vi "Main.vi"() -> ()   [LabVIEW 2020]
uses:
  _controls/_VIWiresData.ctl
  _queue/QueueData.ctl
  _queue/State.ctl
panel:
  in  "Info2 2":string="Step 3: Enjoy!\nLength in cm is calculated assuming 1cm = 16 pixels."
  out "Total wires length (m)":dbl format="%.2f"
  out "Total wires length (pix)":dbl
  in  "Info2":string="Step 2: Calculate wires length!\nNote: For a large number of VIs calculations might take a while!"
  in  "Info1":string="Step 1: Load VIs from folder or project"
  in  "CalculateLength":bool
  out "Number of VIs":i32
  out "VIsData":T1[](array[typedef])
  in  "Stop":bool
  in  "SelectProject":bool
  in  "SelectFolder":bool
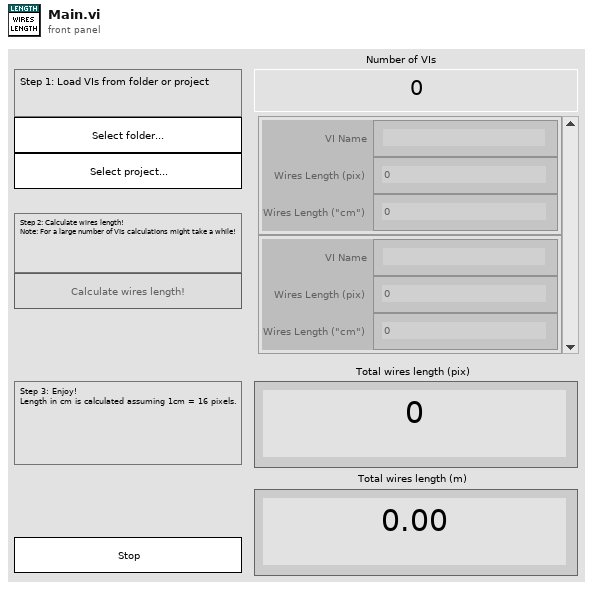
[diagram p1: front panel]
types:
  T1 = typedef "_VIWiresData.ctl" = cluster{"VI Name":string, "Wires Length (pix)":dbl, "Wires Length (\"cm\")":dbl}
  T2 = typedef "QueueData.ctl" = cluster{"State":T3, "Data":variant}
  T3 = typedef "State.ctl" = enum16{"Stop", "LoadFromFolder", "LoadFromProject", "ProcessVIsNames", "AnalyzeVIs"}
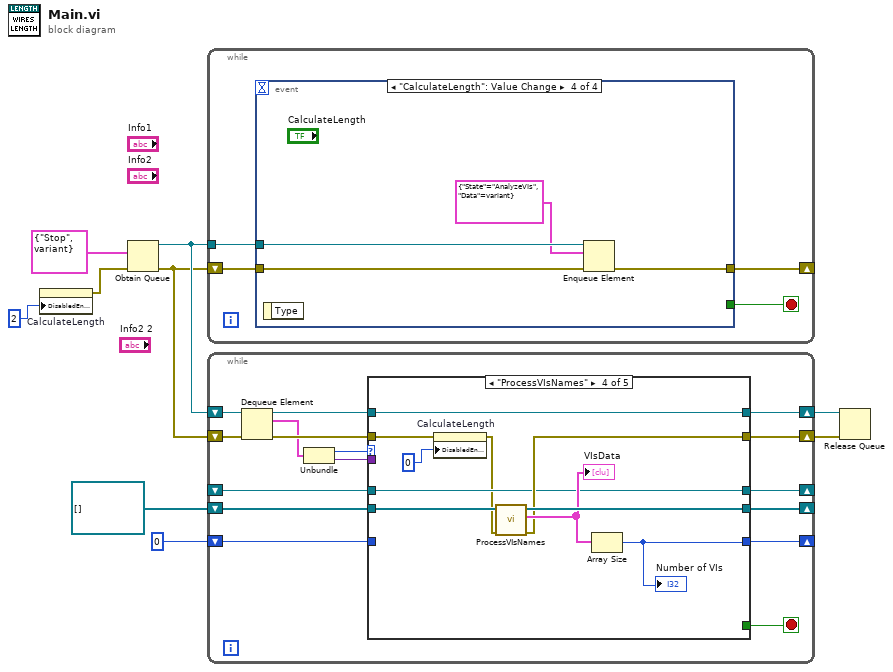
[diagram p0: block diagram]
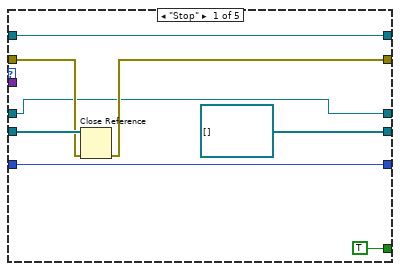
[diagram p2: hidden frame]
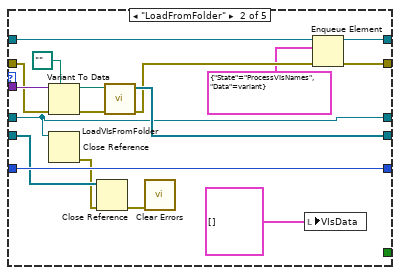
[diagram p3: hidden frame]
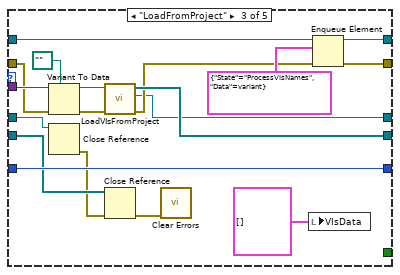
[diagram p4: hidden frame]
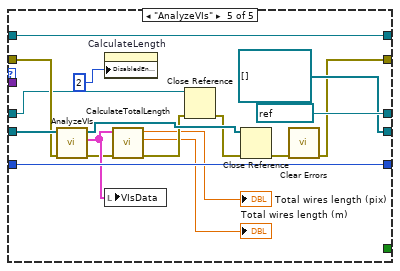
[diagram p5: hidden frame]
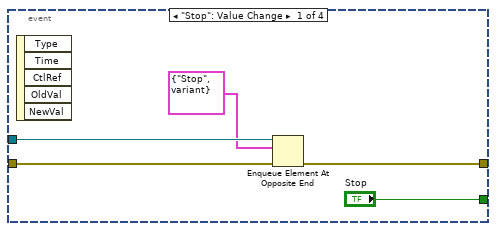
[diagram p6: hidden frame]
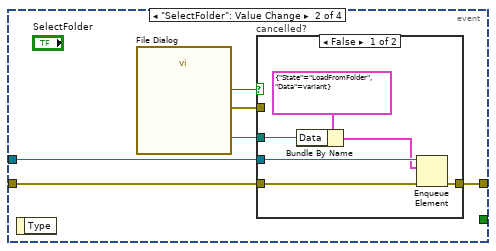
[diagram p7: hidden frame]
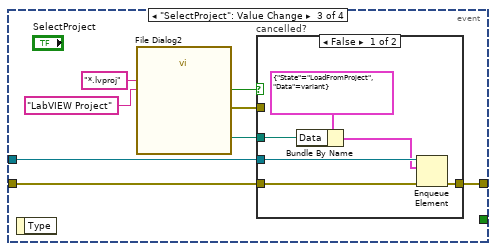
[diagram p9: hidden frame]
diagram:
  n1 = property on="CalculateLength" class="Bool"("DisabledEnum"=2) -> (error out=w1:errorcluster)  [unwired: 2 in, 1 out]
  n2 = Obtain Queue(element data type=T2 {"State"=enum."Stop", "Data"=variant} ("QueueData"), error in (no error)=w1) -> (queue out=w8:refnum<queue>, error out=w7:errorcluster)  [unwired: 3 in, 1 out]
  n3 = while {
    tunnel: w8 -> [w12]
    shift-right: [w10] -> _
    shift-left: w7 -> [w11]
    stop <- w13 stop-if-true
    n4 = event shown="[3] \"CalculateLength\": Value Change" {
      selector: _ -> [_ _ _ _]
      dyn-events: _ -> [_ _ _ _]
      timeout: _ -> [_ _ _ _]
      tunnel: ["Stop" _ _ _] -> w13
      tunnel: w12 -> [w15 w22 w37 w48]
      tunnel: w11 -> [w17 w24 w39 w50]
      tunnel: [w16 w23 w38 w49] -> w10
      event "Stop": Value Change {
        n5 = event-data() -> ()  [unwired: 1 in, 5 out]
        n6 = Enqueue Element At Opposite End(queue=w15, element=T2 {"State"=enum."Stop", "Data"=variant}, error in (no error)=w17) -> (error out=w16:errorcluster)  [unwired: 1 in, 2 out]
      }
      event "SelectFolder": Value Change {
        n7 = event-data() -> ()  [unwired: 1 in, 1 out]
        n8 = call "File Dialog"() -> ("selected path"=w21:path, "cancelled"=w20:bool, "error out"=w19:errorcluster)  [unwired: 12 in, 1 out]
        n9 = case "cancelled?" shown="False" w20 {
          tunnel: w24 -> [w30 w31]
          tunnel: [w29 w31] -> w23
          tunnel: w22 -> [w28 _]
          tunnel: w21 -> [w26 _]
          tunnel: w19 -> [_ _]
          frame False {
            n10 = Bundle By Name(cluster=T2 {"State"=enum."LoadFromFolder", "Data"=variant} ("element"), "Data"=w26) -> (w25:T2)
            n11 = Enqueue Element(queue=w28, element=w25, error in (no error)=w30) -> (error out=w29:errorcluster)  [unwired: 1 in, 2 out]
          }
          frame True {
          }
        }
      }
      event "SelectProject": Value Change {
        n12 = event-data() -> ()  [unwired: 1 in, 1 out]
        n13 = call "File Dialog2"("pattern (all files)"="*.lvproj", "pattern label"="LabVIEW Project") -> ("selected path"=w36:path, "cancelled"=w35:bool, "error out"=w33:errorcluster)  [unwired: 10 in, 1 out]
        n14 = case "cancelled?" shown="False" w35 {
          tunnel: w39 -> [w45 w46]
          tunnel: [w44 w46] -> w38
          tunnel: w37 -> [w43 _]
          tunnel: w36 -> [w41 _]
          tunnel: w33 -> [_ _]
          frame False {
            n15 = Bundle By Name(cluster=T2 {"State"=enum."LoadFromProject", "Data"=variant} ("element"), "Data"=w41) -> (w40:T2)
            n16 = Enqueue Element(queue=w43, element=w40, error in (no error)=w45) -> (error out=w44:errorcluster)  [unwired: 1 in, 2 out]
          }
          frame True {
          }
        }
      }
      event "CalculateLength": Value Change {
        n17 = event-data() -> ()  [unwired: 1 in, 1 out]
        n18 = Enqueue Element(queue=w48, element=T2 {"State"=enum."AnalyzeVIs", "Data"=variant}, error in (no error)=w50) -> (error out=w49:errorcluster)  [unwired: 1 in, 2 out]
      }
    }
  }
  n19 = while {
    shift-right: [w59] -> w6
    shift-left: w7 -> [w65]
    shift-right: [w57] -> w5
    shift-left: w8 -> [w66]
    shift-right: [w56] -> _
    shift-left: refnum<vi>[] [] ("VIs out") -> [w55]
    shift-right: [w54] -> _
    shift-left: 0 -> [w53]
    shift-right: [w52] -> _
    shift-left: _ -> [w51]
    stop <- w58 stop-if-true
    n20 = Dequeue Element(queue=w66, error in (no error)=w65) -> (queue out=w64:refnum<queue>, element=w62:T2, error out=w63:errorcluster)  [unwired: 1 in, 1 out]
    n21 = Unbundle(w62) -> ("State"=w61:T3, "Data"=w60:variant)
    n22 = case shown="\"ProcessVIsNames\"" w61 {
      tunnel: w64 -> [w73 w85 w102 w115 w136]
      tunnel: w63 -> [w71 w90 w108 w112 w133]
      tunnel: w60 -> [_ w91 w109 _ _]
      tunnel: [w70 w83 w99 w116 w120] -> w59
      tunnel: [TRUE _ _ _ _] -> w58
      tunnel: [w73 w82 w101 w115 w136] -> w57
      tunnel: [refnum<vi>[] [] ("VIs") w86 w104 w118 refnum<vi>[] [] ("VIs out")] -> w56
      tunnel: w55 -> [w72 w77 w94 w119 w134]
      tunnel: [w68 w80 w98 w114 w135] -> w54
      tunnel: w53 -> [w68 w80 w98 _ w135]
      tunnel: [w67 w78 w96 w113 refnum<vi> refnum ("Project")] -> w52
      tunnel: w51 -> [w67 w78 w95 w113 w131]
      frame "Stop" {
        n23 = Close Reference(reference=w72, error in (no error)=w71) -> (error out=w70:errorcluster)
      }
      frame "LoadFromFolder" {
        n24 = Variant To Data(error in=w90, type=path "", Variant=w91) -> (data=w88:path, error out=w87:errorcluster)
        n25 = Close Reference(reference=w78) -> (error out=w76:errorcluster)  [unwired: 1 in]
        n26 = Close Reference(reference=w77, error in (no error)=w76) -> (error out=w75:errorcluster)
        n27 = call "LoadVIsFromFolder.vi"("error in (no error)"=w87, "FolderPath"=w88) -> ("error out"=w84:errorcluster, "VIs"=w86:refnum<vi>[])  [unwired: 8 in]
        n28 = call <vilib>:"Clear Errors.vi"("error in (no error)"=w75) -> ()  [unwired: 5 in, 2 out]
        n29 = local write "VIsData"(T1[] [] ("VIsData")) -> ()
        n30 = Enqueue Element(queue=w85, element=T2 {"State"=enum."ProcessVIsNames", "Data"=variant}, error in (no error)=w84) -> (queue out=w82:refnum<queue>, error out=w83:errorcluster)  [unwired: 1 in, 1 out]
      }
      frame "LoadFromProject" {
        n31 = Variant To Data(error in=w108, type=path "", Variant=w109) -> (data=w106:path, error out=w105:errorcluster)
        n32 = Close Reference(reference=w95) -> (error out=w93:errorcluster)  [unwired: 1 in]
        n33 = call "LoadVIsFromProject.vi"("error in (no error)"=w105, "ProjectPath"=w106) -> ("error out"=w100:errorcluster, "Project"=w96:refnum<vi>, "VIs"=w104:refnum<vi>[])  [unwired: 7 in]
        n34 = Close Reference(reference=w94, error in (no error)=w93) -> (error out=w92:errorcluster)
        n35 = call <vilib>:"Clear Errors.vi"("error in (no error)"=w92) -> ()  [unwired: 5 in, 2 out]
        n36 = local write "VIsData"(T1[] [] ("VIsData")) -> ()
        n37 = Enqueue Element(queue=w102, element=T2 {"State"=enum."ProcessVIsNames", "Data"=variant}, error in (no error)=w100) -> (queue out=w101:refnum<queue>, error out=w99:errorcluster)  [unwired: 1 in, 1 out]
      }
      frame "ProcessVIsNames" {
        n38 = property on="CalculateLength" class="Bool"(error in=w112, "DisabledEnum"=0) -> (error out=w111:errorcluster)  [unwired: 1 in, 1 out]
        n39 = call "ProcessVIsNames.vi"("error in (no error)"=w111, "VIs"=w119) -> ("error out"=w116:errorcluster, "VIsData"=w117:T1[], "VIs out"=w118:refnum<vi>[])  [unwired: 7 in]
        "VIsData" <- w117
        n40 = Array Size(array=w117) -> (size(s)=w114:i32)
        "Number of VIs" <- w114
      }
      frame "AnalyzeVIs" {
        n41 = call "AnalyzeVIs.vi"("error in (no error)"=w133, "VIs"=w134) -> ("error out"=w125:errorcluster, "VIsData"=w126:T1[], "VIs out"=w132:refnum<vi>[])  [unwired: 7 in]
        n42 = property on="CalculateLength" class="Bool"("DisabledEnum"=2) -> ()  [unwired: 2 in, 2 out]
        n43 = local write "VIsData"(w126) -> ()
        n44 = call "CalculateTotalLength.vi"("error in (no error)"=w125, "VIsData"=w126) -> ("error out"=w124:errorcluster, "Wires Length (m)"=→"Total wires length (m)":dbl, "Wires Length (pix)"=→"Total wires length (pix)":dbl)  [unwired: 7 in]
        n45 = Close Reference(reference=w131, error in (no error)=w124) -> (error out=w130:errorcluster)
        n46 = Close Reference(reference=w132, error in (no error)=w130) -> (error out=w129:errorcluster)
        n47 = call <vilib>:"Clear Errors.vi"("error in (no error)"=w129) -> ("error out"=w120:errorcluster)  [unwired: 5 in, 1 out]
      }
    }
  }
  n48 = Release Queue(queue=w5, error in (no error)=w6) -> ()  [unwired: 1 in, 3 out]
